vi "CreateQueues.vi"(8 "create semaphore?":bool=TRUE, 9 "create if not found? (T)":bool=TRUE, 10 "client configuration":T3) -> (0 "error out":errorcluster, 3 "output cluster":T1)   [LabVIEW 2014]
uses:
  typedefs/clientConfiguration.ctl
  typedefs/QueueCluster.ctl
  typedefs/clientStatus.ctl
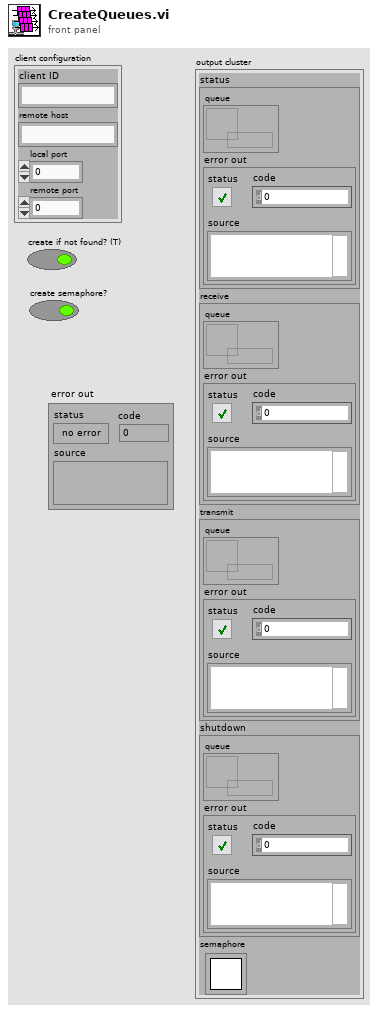
[diagram p1: front panel]
types:
  T1 = typedef "QueueCluster.ctl" = cluster{"status":cluster{"queue":refnum<queue>, "error out":errorcluster}, "receive":cluster{"queue":refnum<queue>, "error out":errorcluster}, "transmit":cluster{"queue":refnum<queue>, "error out":errorcluster}, "shutdown":cluster{"queue":refnum<queue>, "error out":errorcluster}, "semaphore":T2}
  T2 = typedef "Semaphore RefNum" = refnum<k1>
  T3 = typedef "clientConfiguration.ctl" = cluster{"client ID":string, "remote host":string, "local port":u16, "remote port":u16}
  T4 = cluster{"queue out":refnum<queue>, "error out":errorcluster}
  T5 = typedef "clientStatus.ctl" = cluster{"connected":bool, "sent":bool}
  T6 = cluster{"status":cluster{"queue out":refnum<queue>, "error out":errorcluster}, "receive":cluster{"queue out":refnum<queue>, "error out":errorcluster}, "transmit":cluster{"queue out":refnum<queue>, "error out":errorcluster}, "shutdown":cluster{"queue out":refnum<queue>, "error out":errorcluster}, "semaphore":T2}
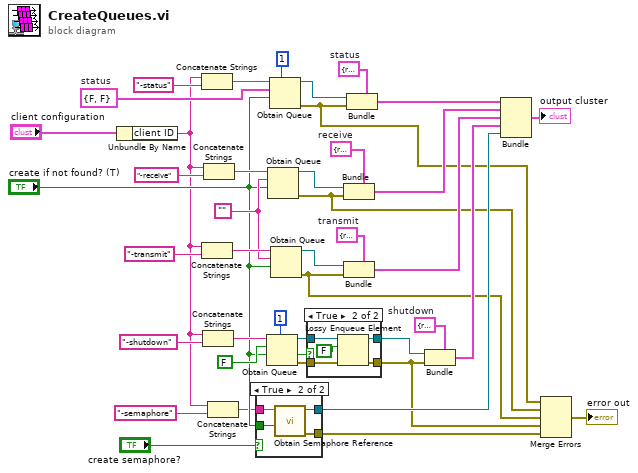
[diagram p0: block diagram]
diagram:
  w20 = T4 {"queue out"=refnum, "error out"={"status"=FALSE, "code"=0, "source"=""}}  # shutdown
  w22 = T4 {"queue out"=refnum, "error out"={"status"=FALSE, "code"=0, "source"=""}}  # transmit
  w24 = T4 {"queue out"=refnum, "error out"={"status"=FALSE, "code"=0, "source"=""}}  # receive
  w27 = T4 {"queue out"=refnum, "error out"={"status"=FALSE, "code"=0, "source"=""}}  # status
  w30 = T5 {"connected"=FALSE, "sent"=FALSE}  # status
  w34 = ""
  n1 = Unbundle By Name("client configuration") -> ("client ID"=w9:string)
  n2 = Concatenate Strings(w9, "-status" ("string")) -> (w40:string)
  n3 = Concatenate Strings(w9, "-transmit" ("string")) -> (w37:string)
  n4 = Concatenate Strings(w9, "-shutdown" ("string")) -> (w42:string)
  n5 = Concatenate Strings(w9, "-receive" ("string")) -> (w35:string)
  n6 = Concatenate Strings(w9, "-semaphore" ("name (unnamed)")) -> (w8:string)
  n7 = case shown="True" "create semaphore?" {
    tunnel: [_ w46] -> w12
    tunnel: "create if not found? (T)" -> [_ w45]
    tunnel: w8 -> [_ w44]
    tunnel: [_ w43] -> w7
    frame False {
    }
    frame True {
      n8 = call <vilib>:"Obtain Semaphore Reference.vi"("create if not found (T)"=w45, "name (unnamed)"=w44) -> ("error out"=w43:errorcluster, "semaphore"=w46:T2)  [unwired: 3 in, 1 out]
    }
  }
  n9 = Obtain Queue(max queue size (-1, unlimited)=1, name (unnamed)=w42, element data type=FALSE, create if not found? (T)="create if not found? (T)") -> (queue out=w21:refnum<queue>, created new?=w13:bool, error out=w14:errorcluster)  [unwired: 1 in]
  n10 = Obtain Queue(name (unnamed)=w35, element data type=w34, create if not found? (T)="create if not found? (T)") -> (queue out=w25:refnum<queue>, error out=w4:errorcluster)  [unwired: 2 in, 1 out]
  n11 = Obtain Queue(max queue size (-1, unlimited)=1, name (unnamed)=w40, element data type=w30, create if not found? (T)="create if not found? (T)") -> (queue out=w28:refnum<queue>, error out=w3:errorcluster)  [unwired: 1 in, 1 out]
  n12 = Obtain Queue(name (unnamed)=w37, element data type=w34, create if not found? (T)="create if not found? (T)") -> (queue out=w23:refnum<queue>, error out=w2:errorcluster)  [unwired: 2 in, 1 out]
  n13 = case shown="True" w13 {
    tunnel: w21 -> [w48 w53]
    tunnel: [w48 w52] -> w15
    tunnel: w14 -> [w47 w51]
    tunnel: [w47 w50] -> w5
    frame False {
    }
    frame True {
      n14 = Lossy Enqueue Element(queue=w53, element=FALSE, error in (no error)=w51) -> (queue out=w52:refnum<queue>, error out=w50:errorcluster)  [unwired: 2 out]
    }
  }
  n15 = Bundle(cluster=w24, "queue out"=w25, "error out"=w4) -> (w19:T4)
  n16 = Bundle(cluster=w22, "queue out"=w23, "error out"=w2) -> (w18:T4)
  n17 = Bundle(cluster=w27, "queue out"=w28, "error out"=w3) -> (w26:T4)
  n18 = Bundle(cluster=w20, "queue out"=w15, "error out"=w5) -> (w17:T4)
  n19 = Bundle("status"=w26, "receive"=w19, "transmit"=w18, "shutdown"=w17, "semaphore"=w12) -> (→"output cluster":T6)  [unwired: 1 in]
  n20 = Merge Errors(w3, w4, w2, w5, w7) -> (→"error out":errorcluster)
